vi "myRIO_BRig_Host_formatData_generic.vi"(8 "input_error":errorcluster, 10 "input_newPath":string, 11 "input_origPath":string) -> (0 "output_error":errorcluster)   [LabVIEW 2014]
uses:
  <vilib>/Utility/file.llb/Read From Spreadsheet File (I64).vi
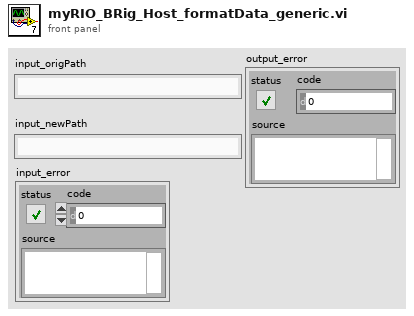
[diagram p1: front panel]
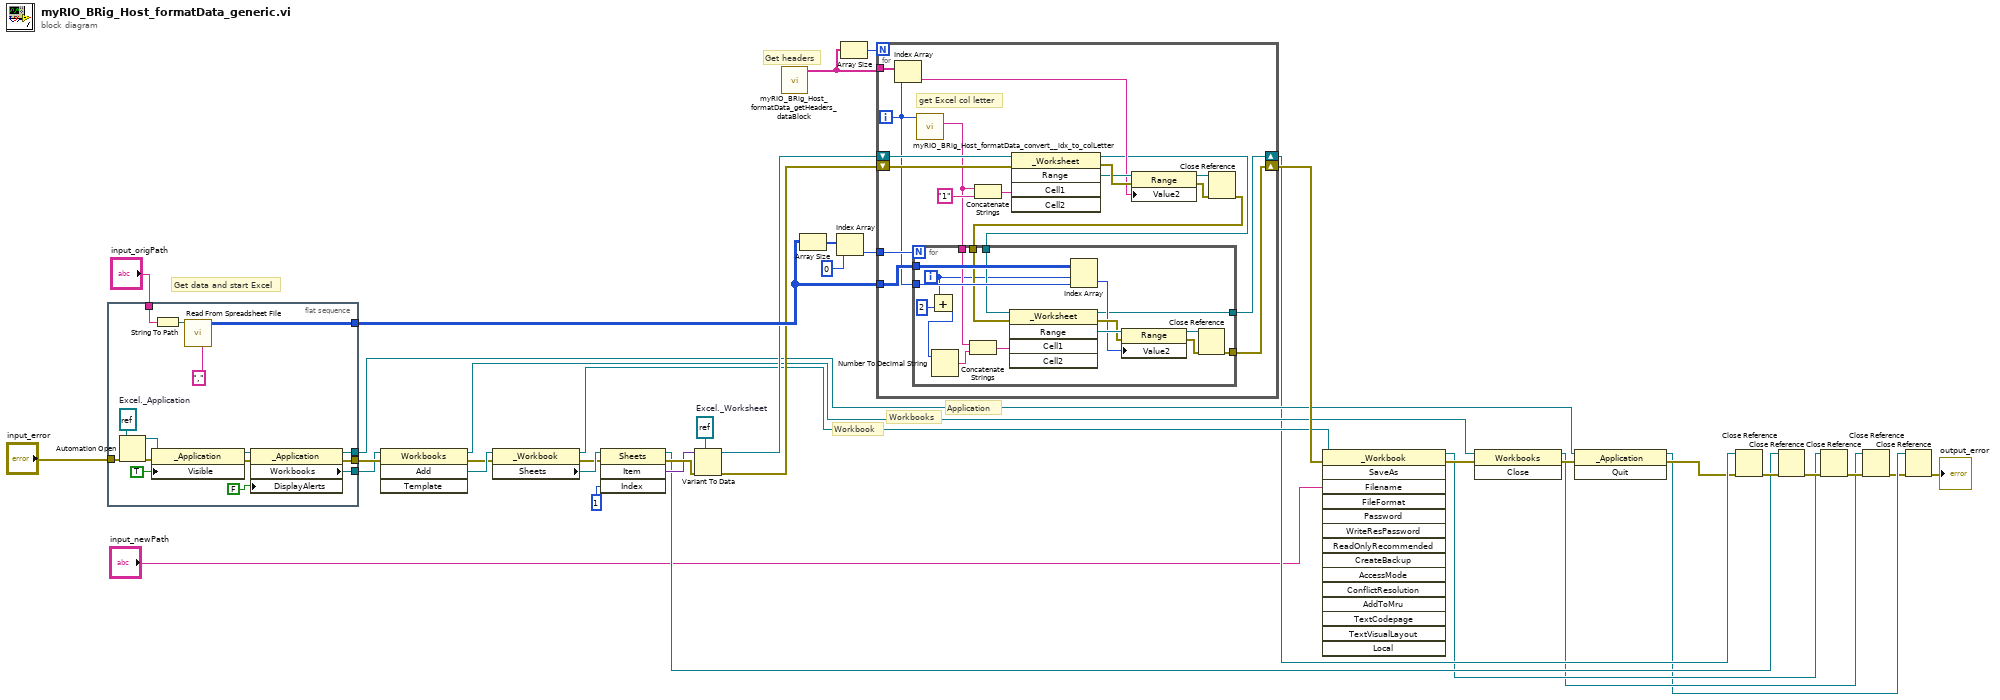
[diagram p0: block diagram]
diagram:
  w28 = refnum<k7> refnum  # Excel._Worksheet
  # "Application"
  # "Workbooks"
  # "Workbook"
  # "Get data and start Excel"
  # "Get headers"
  n1 = flat-sequence {
    tunnel: "input_origPath" -> [w44]
    tunnel: [w43] -> w22
    tunnel: [w42] -> w14
    tunnel: [w41] -> w32
    tunnel: [w40] -> w31
    tunnel: "input_error" -> [w39]
    frame #0 {
      w48 = refnum<k7> refnum  # Excel._Application
      n2 = Automation Open(error in (no error)=w39, Automation Refnum=w48) -> (Automation Refnum=w47:refnum<k7>, error out=w46:errorcluster)  [unwired: 2 out]
      n3 = property class="_Application"(reference=w47, error in=w46, "Visible"=TRUE) -> (reference out=w51:refnum<k7>, error out=w49:errorcluster)
      n4 = String To Path(string=w44) -> (path=w53:path)
      n5 = call-poly <vilib>:"Read From Spreadsheet File.vi"("delimiter (\\t)"="," ("delimiter (\\t)"), "file path (dialog if empty)"=w53) -> ("all rows"=w43:i64[][])  [unwired: 5 in, 4 out]
      n6 = property class="_Application"(reference=w51, error in=w49, "DisplayAlerts"=FALSE) -> (reference out=w42:refnum<k7>, error out=w41:errorcluster, "Workbooks"=w40:refnum<k7>)
    }
  }
  n7 = invoke class="Workbooks" method="Add"(reference=w31, error in=w32) -> (reference out=w15:refnum<k7>, error out=w34:errorcluster, "Add"=w35:refnum<k7>)  [unwired: 2 in, 1 out]
  n8 = property class="_Workbook"(reference=w35, error in=w34) -> (reference out=w18:refnum<k7>, error out=w36:errorcluster, "Sheets"=w37:refnum<k7>)
  n9 = invoke class="Sheets" method="Item"(reference=w37, error in=w36, "Index"=1) -> (reference out=w11:refnum<k7>, error out=w30:errorcluster, "Item"=w29:variant)  [unwired: 1 in, 1 out]
  n10 = Variant To Data(error in=w30, type=w28, Variant=w29) -> (data=w21:refnum<k7>, error out=w20:errorcluster)
  n11 = call "myRIO_BRig_Host_formatData_getHeaders_dataBlock.vi"() -> ("output_stringArray_dataBlock"=w26:string[])  [unwired: 11 in]
  n12 = Array Size(array=w22) -> (size(s)=w25:i32[])
  n13 = Index Array(array=w25, index=0) -> (element=w23:i32)
  n14 = Array Size(array=w26) -> (size(s)=w27:i32)
  n15 = for {
    N: w27 -> [_]
    tunnel: w26 -> [w71]
    shift-right: [w58] -> w13
    shift-left: w21 -> [w69]
    shift-right: [w59] -> w19
    shift-left: w20 -> [w68]
    tunnel: w22 -> [w60]
    tunnel: w23 -> [w61]
    i -> [w55]
    # "get Excel col letter"
    n16 = Index Array(array=w71, index=w55) -> (element=w64:string)
    n17 = call "myRIO_BRig_Host_formatData_convert__idx_to_colLetter.vi"("input_idx"=w55) -> ("output_colLetter"=w54:string)  [unwired: 10 in]
    n18 = Concatenate Strings(w54, "1" ("string")) -> (w66:string)
    n19 = invoke class="_Worksheet" method="Range"(reference=w69, error in=w68, "Cell1"=w66) -> (reference out=w56:refnum<k7>, error out=w67:errorcluster, "Range"=w65:refnum<k7>)  [unwired: 2 in, 2 out]
    n20 = property class="Range"(reference=w65, error in=w67, "Value2"=w64) -> (reference out=w63:refnum<k7>, error out=w62:errorcluster)
    n21 = Close Reference(reference=w63, error in (no error)=w62) -> (error out=w57:errorcluster)
    n22 = for {
      N: w61 -> [_]
      tunnel: w55 -> [w82]
      tunnel: w60 -> [w83]
      tunnel: w54 -> [w80]
      tunnel: [w79] -> w59
      tunnel: [w78] -> w58
      tunnel: w57 -> [w77]
      tunnel: w56 -> [w76]
      i -> [w75]
      n23 = Add(x=w75, y=2 ("string")) -> (x+y=w72:i32)
      n24 = Number To Decimal String(number=w72) -> (decimal integer string=w73:string)  [unwired: 1 in]
      n25 = Concatenate Strings(w80, w73) -> (w88:string)
      n26 = invoke class="_Worksheet" method="Range"(reference=w76, error in=w77, "Cell1"=w88) -> (reference out=w78:refnum<k7>, error out=w86:errorcluster, "Range"=w87:refnum<k7>)  [unwired: 2 in, 2 out]
      n27 = Index Array(array=w83, index (row)=w75, index (col)=w82) -> (element=w81:i64)
      n28 = property class="Range"(reference=w87, error in=w86, "Value2"=w81) -> (reference out=w85:refnum<k7>, error out=w84:errorcluster)
      n29 = Close Reference(reference=w85, error in (no error)=w84) -> (error out=w79:errorcluster)
    }
  }
  n30 = invoke class="_Workbook" method="SaveAs"(reference=w18, error in=w19, "Filename"="input_newPath") -> (reference out=w7:refnum<k7>, error out=w17:errorcluster)  [unwired: 12 in, 13 out]
  n31 = invoke class="Workbooks" method="Close"(reference=w15, error in=w17) -> (reference out=w6:refnum<k7>, error out=w16:errorcluster)  [unwired: 1 in, 1 out]
  n32 = invoke class="_Application" method="Quit"(reference=w14, error in=w16) -> (reference out=w5:refnum<k7>, error out=w10:errorcluster)  [unwired: 1 in, 1 out]
  n33 = Close Reference(reference=w13, error in (no error)=w10) -> (error out=w12:errorcluster)
  n34 = Close Reference(reference=w11, error in (no error)=w12) -> (error out=w9:errorcluster)
  n35 = Close Reference(reference=w7, error in (no error)=w9) -> (error out=w8:errorcluster)
  n36 = Close Reference(reference=w6, error in (no error)=w8) -> (error out=w3:errorcluster)
  n37 = Close Reference(reference=w5, error in (no error)=w3) -> (error out=→"output_error":errorcluster)
